vi "CmdExe.ExecCmd with Timeout and Abort.vi"(5 "Wait until completion? (T)":bool=TRUE, 6 "Timeout ms(-1)":i32=-1, 7 "Run minimized? (T)":bool=TRUE, 8 "error in":errorcluster, 9 "Arguements":string, 10 "Executable":string, 11 "Working Dir":path=path "") -> (0 "error out":errorcluster, 1 "Timed Out":bool, 2 "STD ERR":string, 3 "STD OUT":string, 4 "Aborted":bool)   [LabVIEW 2019]
panel:
  out "return code":i32
  out "Task Killed":bool
  # "Launch Cmd Exe"
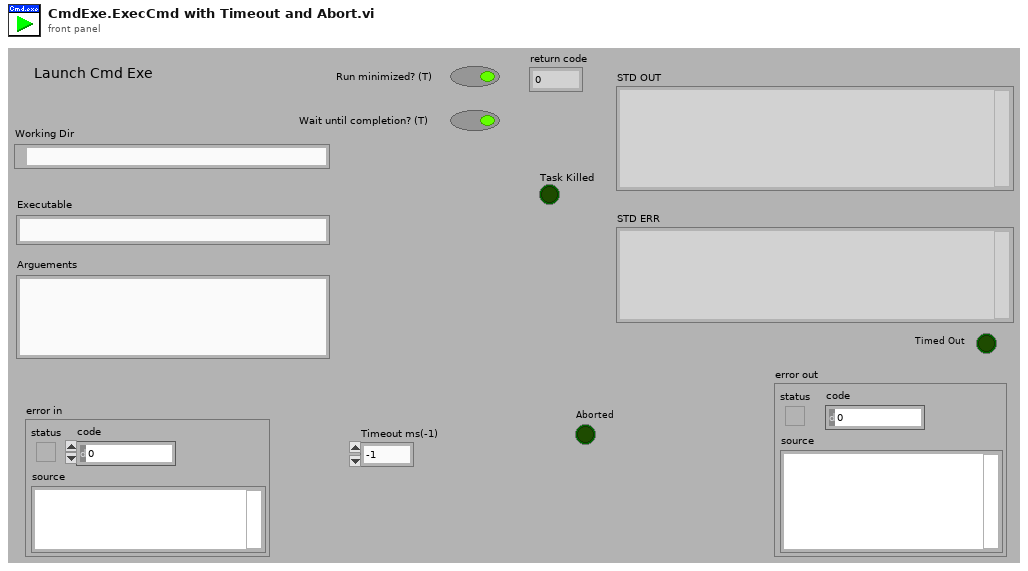
[diagram p1: front panel]
types:
  T1 = cluster{"Ref":refnum<vi>, "Abort":bool, "Timeout":bool, "Cmd":string, "Exe":string, "StdErr":string}
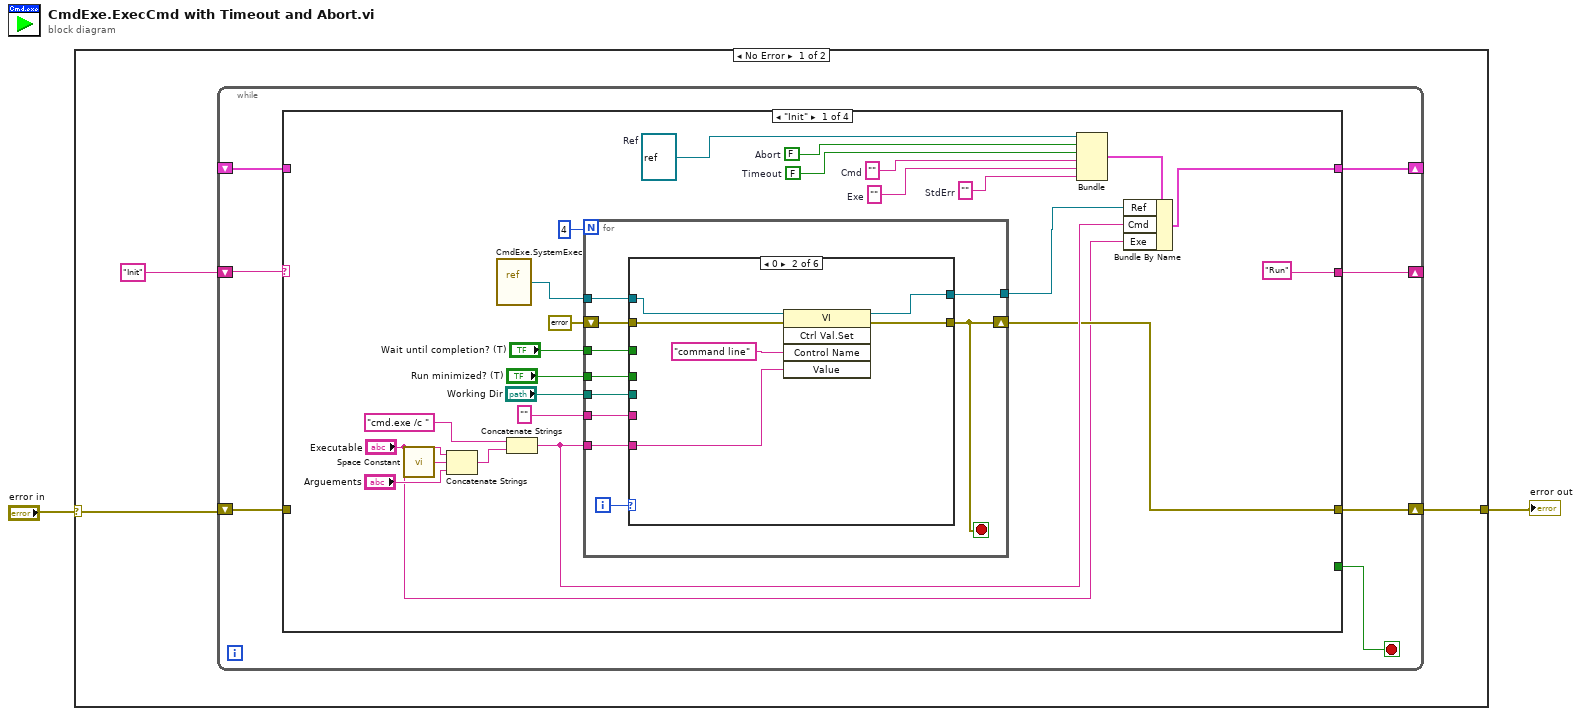
[diagram p0: block diagram]
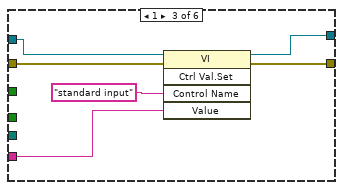
[diagram p3: hidden frame]
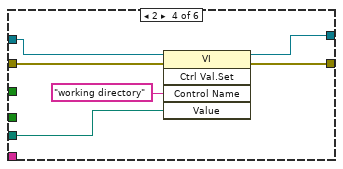
[diagram p4: hidden frame]
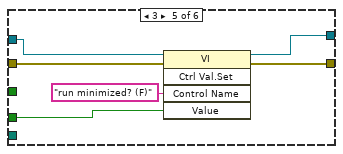
[diagram p5: hidden frame]
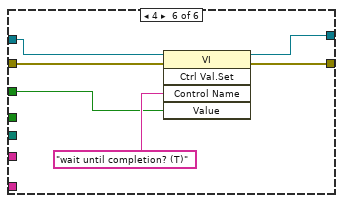
[diagram p6: hidden frame]
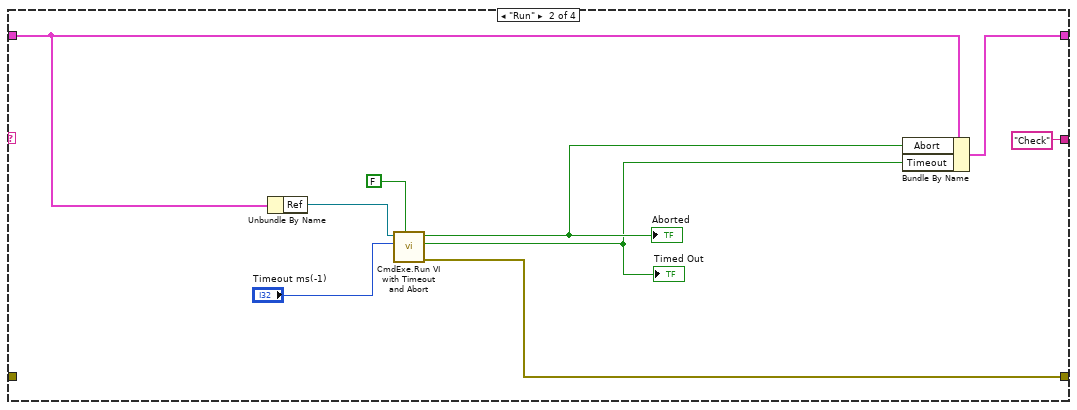
[diagram p7: hidden frame]
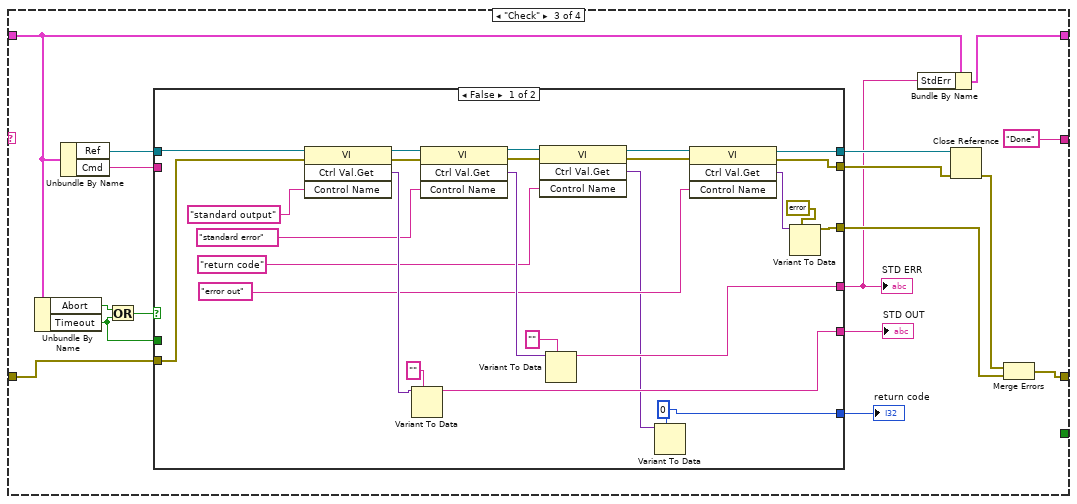
[diagram p8: hidden frame]
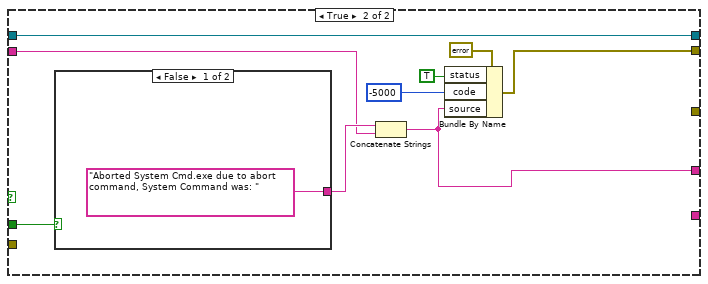
[diagram p9: hidden frame]
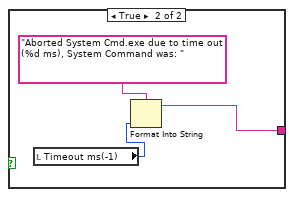
[diagram p10: hidden frame]
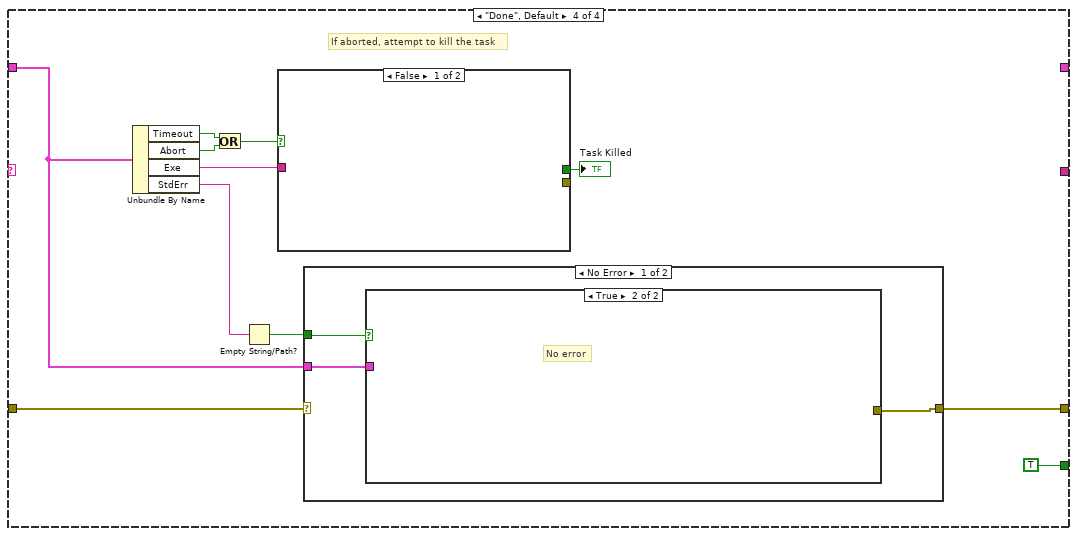
[diagram p11: hidden frame]
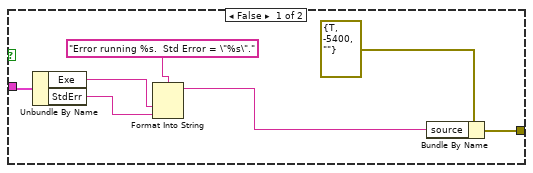
[diagram p12: hidden frame]
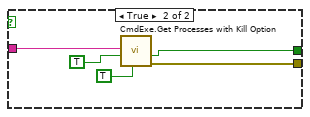
[diagram p14: hidden frame]
diagram:
  n1 = case shown="No Error" "error in" {
    selector: "error in" -> [w4 w170]
    tunnel: [w3 w170] -> w1
    frame No Error {
      n2 = while {
        shift-right: [w10] -> _
        shift-left: _ -> [w11]
        shift-right: [w9] -> _
        shift-left: "Init" -> [w12]
        shift-right: [w7] -> w3
        shift-left: w4 -> [w8]
        stop <- w6 stop-if-true
        n3 = case shown="\"Init\"" w12 {
          tunnel: w11 -> [_ w85 w91 w143]
          tunnel: [w26 w84 w90 _] -> w10
          tunnel: ["Run" "Check" "Done" _] -> w9
          tunnel: [_ _ _ TRUE] -> w6
          tunnel: w8 -> [_ _ w96 w147]
          tunnel: [w21 w81 w94 w144] -> w7
          frame "Init" {
            w13 = ""  # StdErr
            w16 = ""  # Exe
            w23 = ""  # Cmd
            w24 = FALSE  # Timeout
            w25 = FALSE  # Abort
            w30 = refnum<vi> refnum  # Ref
            n4 = call <vilib>:"Space Constant.vi"() -> ("String"=w17:string)
            n5 = Concatenate Strings("Executable", w17, "Arguements") -> (w18:string)
            n6 = vi-ref "CmdExe.SystemExec.vi"() -> (w36:refnum<vi>)
            n7 = Concatenate Strings("cmd.exe /c ", w18) -> (w22:string)
            n8 = for {
              N: 4 -> [_]
              shift-right: [w37] -> w21
              shift-left: errorcluster {"status"=FALSE, "code"=0, "source"=""} ("error constant") -> [w46]
              tunnel: w36 -> [w45]
              tunnel: [w44] -> w28
              tunnel: w22 -> [w42]
              tunnel: "" -> [w41]
              tunnel: "Working Dir" -> [w40]
              tunnel: "Run minimized? (T)" -> [w39]
              tunnel: "Wait until completion? (T)" -> [w38]
              i -> [w43]
              stop <- w37 stop-if-true
              n9 = case shown="0" w43 {
                tunnel: w46 -> [w47 w53 w59 w65 w71 w77]
                tunnel: w45 -> [w48 w52 w58 w64 w70 w76]
                tunnel: [w47 w51 w57 w63 w69 w75] -> w37
                tunnel: [w48 w50 w56 w62 w68 w74] -> w44
                tunnel: w42 -> [_ w49 _ _ _ _]
                tunnel: w41 -> [_ _ w55 _ _ _]
                tunnel: w40 -> [_ _ _ w61 _ _]
                tunnel: w39 -> [_ _ _ _ w67 _]
                tunnel: w38 -> [_ _ _ _ _ w73]
                frame 99, Default {
                }
                frame 0 {
                  n10 = invoke class="VI" method="Ctrl Val.Set"(reference=w52, error in=w53, "Control Name"="command line", "Value"=w49) -> (reference out=w50:refnum<vi>, error out=w51:errorcluster)  [unwired: 1 in, 3 out]
                }
                frame 1 {
                  n11 = invoke class="VI" method="Ctrl Val.Set"(reference=w58, error in=w59, "Control Name"="standard input", "Value"=w55) -> (reference out=w56:refnum<vi>, error out=w57:errorcluster)  [unwired: 1 in, 3 out]
                }
                frame 2 {
                  n12 = invoke class="VI" method="Ctrl Val.Set"(reference=w64, error in=w65, "Control Name"="working directory", "Value"=w61) -> (reference out=w62:refnum<vi>, error out=w63:errorcluster)  [unwired: 1 in, 3 out]
                }
                frame 3 {
                  n13 = invoke class="VI" method="Ctrl Val.Set"(reference=w70, error in=w71, "Control Name"="run minimized? (F)", "Value"=w67) -> (reference out=w68:refnum<vi>, error out=w69:errorcluster)  [unwired: 1 in, 3 out]
                }
                frame 4 {
                  n14 = invoke class="VI" method="Ctrl Val.Set"(reference=w76, error in=w77, "Control Name"="wait until completion? (T)", "Value"=w73) -> (reference out=w74:refnum<vi>, error out=w75:errorcluster)  [unwired: 1 in, 3 out]
                }
              }
            }
            n15 = Bundle("Ref"=w30, "Abort"=w25, "Timeout"=w24, "Cmd"=w23, "Exe"=w16, "StdErr"=w13) -> (w27:T1)  [unwired: 1 in]
            n16 = Bundle By Name(cluster=w27, "Ref"=w28, "Cmd"=w22, "Exe"="Executable") -> (w26:T1)
          }
          frame "Run" {
            n17 = Unbundle By Name(w85) -> ("Ref"=w80:refnum<vi>)
            n18 = call "CmdExe.Run VI with Timeout and Abort.vi"("Close Ref"=FALSE, "Timeout ms(-1)"="Timeout ms(-1)", "VI Refnum"=w80) -> ("error out"=w81:errorcluster, "Timeout"=w82:bool, "Abort"=w83:bool)  [unwired: 6 in]
            "Timed Out" <- w82
            "Aborted" <- w83
            n19 = Bundle By Name(cluster=w85, "Abort"=w83, "Timeout"=w82) -> (w84:T1)
          }
          frame "Check" {
            n20 = Unbundle By Name(w91) -> ("Abort"=w103:bool, "Timeout"=w97:bool)
            n21 = Unbundle By Name(w91) -> ("Ref"=w102:refnum<vi>, "Cmd"=w101:string)
            n22 = Or(x=w103, y=w97) -> (x .or. y?=w104:bool)
            n23 = case shown="False" w104 {
              tunnel: w102 -> [w129 w138]
              tunnel: [w117 w138] -> w99
              tunnel: [w116 w135] -> w98
              tunnel: [w120 w133] -> w89
              tunnel: [w119 _] -> w100
              tunnel: w101 -> [_ w131]
              tunnel: w97 -> [_ w130]
              tunnel: w96 -> [w118 _]
              tunnel: [w112 _] -> w93
              tunnel: [w105 _] -> w88
              frame False {
                w105 = 0 ("return code")
                n24 = invoke class="VI" method="Ctrl Val.Get"(reference=w129, error in=w118, "Control Name"="standard output") -> (reference out=w122:refnum<vi>, error out=w121:errorcluster, "Get Control Value Variant"=w127:variant)  [unwired: 1 in, 1 out]
                n25 = Variant To Data(type="", Variant=w127) -> (data=w119:string)  [unwired: 1 in, 1 out]
                n26 = invoke class="VI" method="Ctrl Val.Get"(reference=w122, error in=w121, "Control Name"="standard error") -> (reference out=w111:refnum<vi>, error out=w110:errorcluster, "Get Control Value Variant"=w124:variant)  [unwired: 1 in, 1 out]
                n27 = invoke class="VI" method="Ctrl Val.Get"(reference=w111, error in=w110, "Control Name"="return code") -> (reference out=w108:refnum<vi>, error out=w109:errorcluster, "Get Control Value Variant"=w106:variant)  [unwired: 1 in, 1 out]
                n28 = Variant To Data(type="", Variant=w124) -> (data=w120:string)  [unwired: 1 in, 1 out]
                n29 = Variant To Data(type=w105, Variant=w106) -> ()  [unwired: 1 in, 2 out]
                n30 = invoke class="VI" method="Ctrl Val.Get"(reference=w108, error in=w109, "Control Name"="error out") -> (reference out=w117:refnum<vi>, error out=w116:errorcluster, "Get Control Value Variant"=w114:variant)  [unwired: 1 in, 1 out]
                n31 = Variant To Data(type=errorcluster {"status"=FALSE, "code"=0, "source"=""} ("error constant"), Variant=w114) -> (data=w112:errorcluster)  [unwired: 1 in, 1 out]
              }
              frame True {
                n32 = case shown="False" w130 {
                  tunnel: ["Aborted System Cmd.exe due to abort command, System Command was: " ("source") w141] -> w134
                  frame False {
                  }
                  frame True {
                    n33 = local read "Timeout ms(-1)"() -> (w140:i32)
                    n34 = Format Into String(format string="Aborted System Cmd.exe due to time out (%d ms), System Command was: " ("source"), w140) -> (resulting string=w141:string)  [unwired: 2 in, 1 out]
                  }
                }
                n35 = Concatenate Strings(w134, w131) -> (w133:string)
                n36 = Bundle By Name(cluster=errorcluster {"status"=FALSE, "code"=0, "source"=""} ("error constant"), "status"=TRUE ("Wait Until Done"), "code"=-5000, "source"=w133) -> (w135:errorcluster)
              }
            }
            "STD ERR" <- w89
            "STD OUT" <- w100
            "return code" <- w88
            n37 = Bundle By Name(cluster=w91, "StdErr"=w89) -> (w90:T1)
            n38 = Close Reference(reference=w99, error in (no error)=w98) -> (error out=w95:errorcluster)
            n39 = Merge Errors(w95, w93) -> (w94:errorcluster)
          }
          frame "Done", Default {
            # "If aborted, attempt to kill the task"
            n40 = Unbundle By Name(w143) -> ("Timeout"=w151:bool, "Abort"=w150:bool, "Exe"=w152:string, "StdErr"=w145:string)
            n41 = Or(x=w151, y=w150) -> (x .or. y?=w149:bool)
            n42 = Empty String/Path?(string/path=w145) -> (empty?=w146:bool)
            n43 = case shown="False" w149 {
              tunnel: w152 -> [_ w169]
              tunnel: [_ w166] -> _
              tunnel: [_ w165] -> w148
              frame False {
              }
              frame True {
                n44 = call "CmdExe.Get Processes with Kill Option.vi"("Kill Only 1 Instance"=TRUE, "Kill Task"=TRUE, "Process Name"=w169) -> ("Error Out"=w166:errorcluster, "Task Killed"=w165:bool)  [unwired: 5 in, 2 out]
              }
            }
            "Task Killed" <- w148
            n45 = case shown="No Error" w147 {
              selector: w147 -> [_ w164]
              tunnel: w146 -> [w156 _]
              tunnel: [w154 w164] -> w144
              tunnel: w143 -> [w155 _]
              frame No Error {
                n46 = case shown="True" w156 {
                  tunnel: w155 -> [w163 _]
                  tunnel: [w157 _] -> w154
                  frame False {
                    n47 = Unbundle By Name(w163) -> ("Exe"=w160:string, "StdErr"=w159:string)
                    n48 = Format Into String(format string="Error running %s.  Std Error = \"%s\".", w160, w159) -> (resulting string=w158:string)  [unwired: 2 in, 1 out]
                    n49 = Bundle By Name(cluster=errorcluster {"status"=TRUE, "code"=-5400, "source"=""} ("error constant"), "source"=w158) -> (w157:errorcluster)
                  }
                  frame True {
                    # "No error"
                  }
                }
              }
              frame Error {
              }
            }
          }
        }
      }
    }
    frame Error {
    }
  }
  "error out" <- w1
